vi "Teleop.vi"(10 "Match Info":T2={"Autonomous Elapsed Seconds"=0.0, "TeleOp Elapsed Seconds"=0.0, "Disabled Elapsed Seconds"=0.0, "Visited Autonomous"=FALSE, "Visited TeleOp"=FALSE, "Visited Disabled"=FALSE, "Autonomous Settings"={"Autonomous Style"=enum."Independent", "VI Refnum"=refnum}}, 11 "Call Context":T1) -> ()   [LabVIEW 2018]
doc: "This VI is called for each enabled TeleOp packet received from the DS. It is typically used to read from joysticks and other inputs and update I/O or setpoints for timed control loops. It should complete and return within 20 milliseconds or risk missing DS packets."
uses:
  <vilib>/Rock Robotics/WPI/DriverStation/WPI_DriverStationMatch Info.ctl
  <vilib>/Rock Robotics/WPI/DriverStation/WPI_DriverStationDerivedRobotMode.ctl
  Support Code/Controller Values.ctl
  <vilib>/Rock Robotics/WPI/Utilities/WPI_GetSetVariantRefNum.vi
  <vilib>/Rock Robotics/Network Tables/NT Write Boolean Array.vi
  <vilib>/Rock Robotics/Network Tables/NT Write Numeric Array.vi
panel:
  out "Compressor Running":bool
  out "Enabled":bool
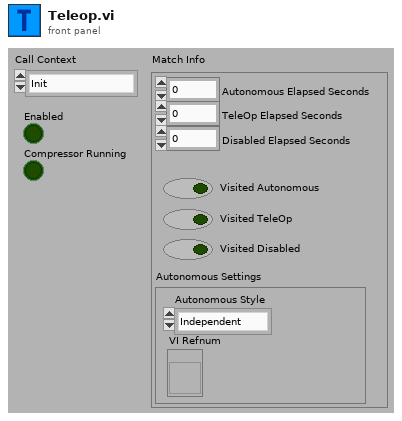
[diagram p1: front panel]
types:
  T1 = typedef "WPI_DriverStationDerivedRobotMode.ctl" = enum16{"Init", "Execute", "Stop"}
  T2 = typedef "WPI_DriverStationMatch Info.ctl" = cluster{"Autonomous Elapsed Seconds":dbl, "TeleOp Elapsed Seconds":dbl, "Disabled Elapsed Seconds":dbl, "Visited Autonomous":bool, "Visited TeleOp":bool, "Visited Disabled":bool, "Autonomous Settings":cluster{"Autonomous Style":enum16{"Iterative", "Independent"}, "VI Refnum":refnum<vi>}}
  T3 = typedef "Controller Values.ctl" = cluster{"Left Joystick Axes ":dbl[], "Right Joystick Axes":dbl[], "Left Joystick Buttons":bool[], "Right Joystick Buttons":bool[], "XBox Axes":dbl[], "XBox Buttons":bool[], "XBox POVs":i16[], "DDR Buttons":bool[]}
  T4 = typedef "WPI_JoystickDevRef.ctl" = cluster{"Device":T5}
  T5 = typedef "WPI_JoystickDeviceEnum.ctl" = enum16{"USB 0", "USB 1", "USB 2", "USB 3", "USB 4", "USB 5"}
  T6 = typedef "WPI_CompressorDevRef.ctl" = cluster{"DevStatus":errorcluster, "Pneumatics Control Module":u8}
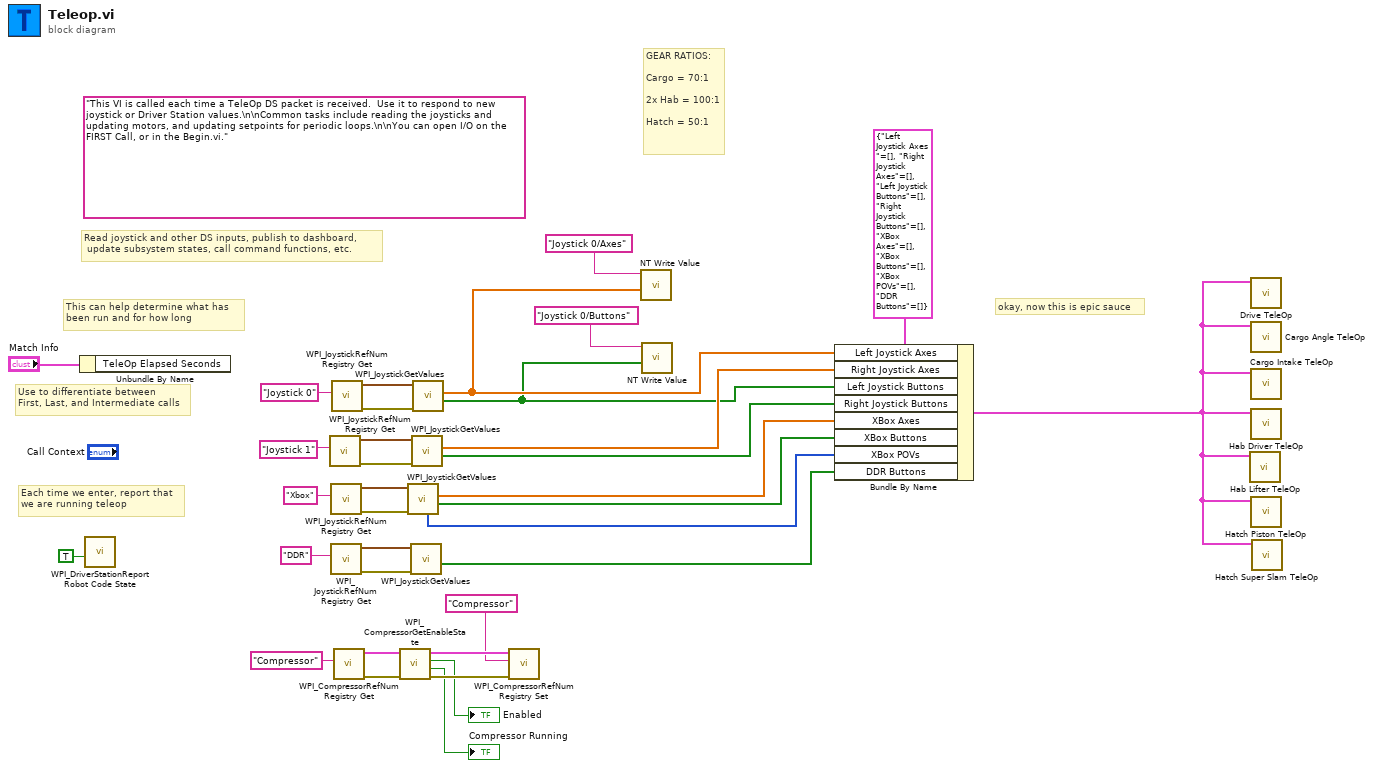
[diagram p0: block diagram]
diagram:
  (unwired) "This VI is called each time a TeleOp DS packet is received.  Use it to respond to new joystick or Driver Station values.\n\nCommon tasks include reading the joysticks and updating motors, and updating setpoints for periodic loops.\n\nYou can open I/O on the FIRST Call, or in the Begin.vi."
  # "GEAR RATIOS:\n\nCargo = 70:1\n\n2x Hab = 100:1\n\nHatch = 50:1"
  # "Each time we enter, report that\nwe are running teleop"
  # "Use to differentiate between\nFirst, Last, and Intermediate calls"
  # "This can help determine what has\nbeen run and for how long"
  # "okay, now this is epic sauce"
  # "Read joystick and other DS inputs, publish to dashboard,\n update subsystem states, call command functions, etc."
  n1 = Unbundle By Name("Match Info") -> ()  [unwired: 1 out]
  n2 = call <vilib>:"WPI_DriverStationReport Robot Code State.vi"("TeleOp"=TRUE ("Autonomous")) -> ()  [unwired: 10 in, 1 out]
  n3 = call <vilib>:"WPI_JoystickRefNum Registry Get.vi"("refnum name"="Joystick 1") -> ("error out"=w26:errorcluster, "JoystickDevRef"=w27:T4)  [unwired: 1 in, 8 out]
  n4 = call <vilib>:"WPI_JoystickRefNum Registry Get.vi"("refnum name"="Xbox") -> ("error out"=w11:errorcluster, "JoystickDevRef"=w22:T4)  [unwired: 1 in, 8 out]
  n5 = call <vilib>:"WPI_JoystickRefNum Registry Get.vi"("refnum name"="DDR") -> ("error out"=w12:errorcluster, "JoystickDevRef"=w24:T4)  [unwired: 1 in, 8 out]
  n6 = call <vilib>:"WPI_JoystickRefNum Registry Get.vi"("refnum name"="Joystick 0") -> ("error out"=w29:errorcluster, "JoystickDevRef"=w32:T4)  [unwired: 1 in, 8 out]
  n7 = call <vilib>:"WPI_CompressorRefNum Registry Get.vi"("refnum name"="Compressor") -> ("error out"=w6:errorcluster, "CompressorDevRef"=w8:T6)  [unwired: 9 in]
  n8 = call <vilib>:"WPI_CompressorGetEnableState.vi"("error in (no error)"=w6, "CompressorDevRef"=w8) -> ("error out"=w5:errorcluster, "Compressor Running"=→"Compressor Running":bool, "Enabled"=→"Enabled":bool, "CompressorDevRef"=w7:T6)  [unwired: 6 in]
  n9 = call <vilib>:"WPI_JoystickGetValues.vi"("error in (no error)"=w11, "JoystickDevRef"=w22) -> ("Buttons"=w16:bool[], "Axes"=w17:dbl[], "POVs"=w15:i16[])  [unwired: 5 in, 2 out]
  n10 = call <vilib>:"WPI_JoystickGetValues.vi"("error in (no error)"=w12, "JoystickDevRef"=w24) -> ("Buttons"=w14:bool[])  [unwired: 5 in, 4 out]
  n11 = call <vilib>:"WPI_JoystickGetValues.vi"("error in (no error)"=w26, "JoystickDevRef"=w27) -> ("Buttons"=w19:bool[], "Axes"=w20:dbl[])  [unwired: 5 in, 3 out]
  n12 = call <vilib>:"WPI_JoystickGetValues.vi"("error in (no error)"=w29, "JoystickDevRef"=w32) -> ("Buttons"=w1:bool[], "Axes"=w21:dbl[])  [unwired: 5 in, 3 out]
  n13 = call <vilib>:"WPI_CompressorRefNum Registry Set.vi"("error in (no error)"=w5, "refnum name"="Compressor", "CompressorDevRef"=w7) -> ()  [unwired: 7 in, 2 out]
  n14 = call-poly <vilib>:"NT Write Value.vi"("Numeric Array"=w21, "Name"="Joystick 0/Axes") -> ()  [unwired: 9 in, 1 out]
  n15 = call-poly <vilib>:"NT Write Value.vi"("Boolean Array"=w1, "Name"="Joystick 0/Buttons") -> ()  [unwired: 9 in, 1 out]
  n16 = Bundle By Name(cluster=T3 {"Left Joystick Axes "=[], "Right Joystick Axes"=[], "Left Joystick Buttons"=[], "Right Joystick Buttons"=[], "XBox Axes"=[], "XBox Buttons"=[], "XBox POVs"=[], "DDR Buttons"=[]} ("Cluster"), "Left Joystick Axes"=w21, "Right Joystick Axes"=w20, "Left Joystick Buttons"=w1, "Right Joystick Buttons"=w19, "XBox Axes"=w17, "XBox Buttons"=w16, "XBox POVs"=w15, "DDR Buttons"=w14) -> (w13:T3)
  n17 = call "Hab Lifter TeleOp.vi"("Controller Values"=w13) -> ()  [unwired: 11 in]
  n18 = call "Drive TeleOp.vi"("Controller Values"=w13) -> ()  [unwired: 11 in]
  n19 = call "Cargo Angle TeleOp.vi"("Controller Values"=w13) -> ()  [unwired: 11 in]
  n20 = call "Cargo Intake TeleOp.vi"("Controller Values"=w13) -> ()  [unwired: 11 in]
  n21 = call "Hab Driver TeleOp.vi"("Controller Values"=w13) -> ()  [unwired: 11 in]
  n22 = call "Hatch Piston TeleOp.vi"("Controller Values"=w13) -> ()  [unwired: 11 in]
  n23 = call "Hatch Super Slam TeleOp.vi"("Controller Values"=w13) -> ()  [unwired: 11 in]
